vi "FAValuesXYZC.vi"(11 "Input":string[](array[string])) -> (3 "Output":string[][](array[string]))   [LabVIEW 2016, in "M1M3SupportEUI_Views.lvlib"]
uses:
  M1M3SupportEUI_Views.lvlib
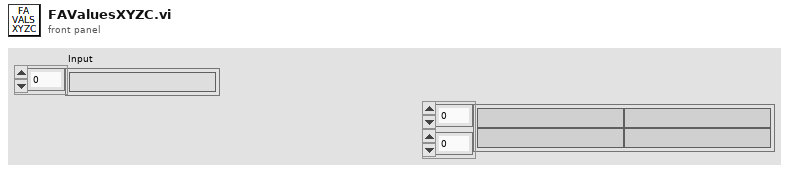
[diagram p1: front panel]
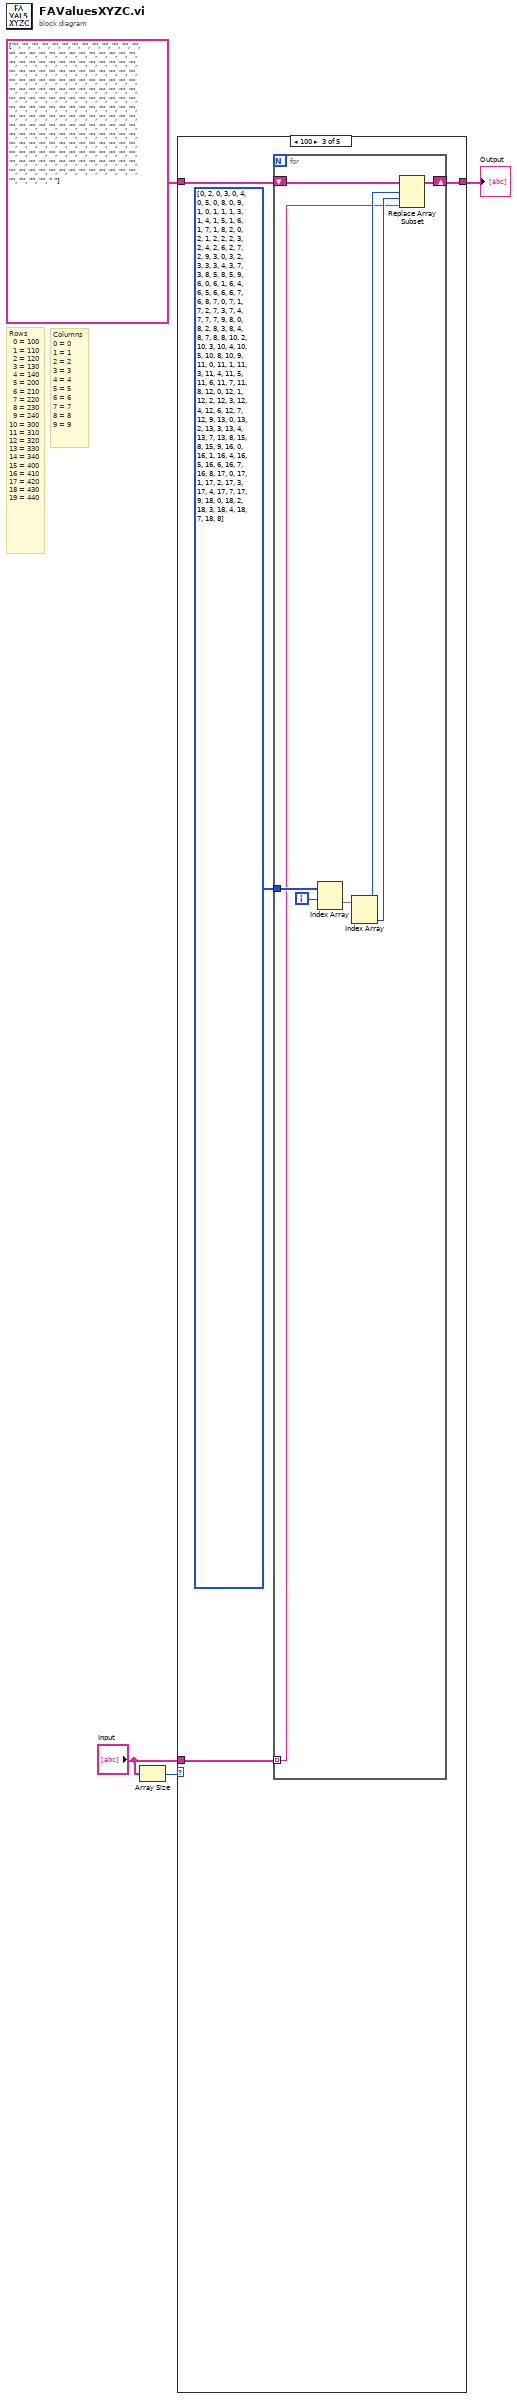
[diagram p0: block diagram]
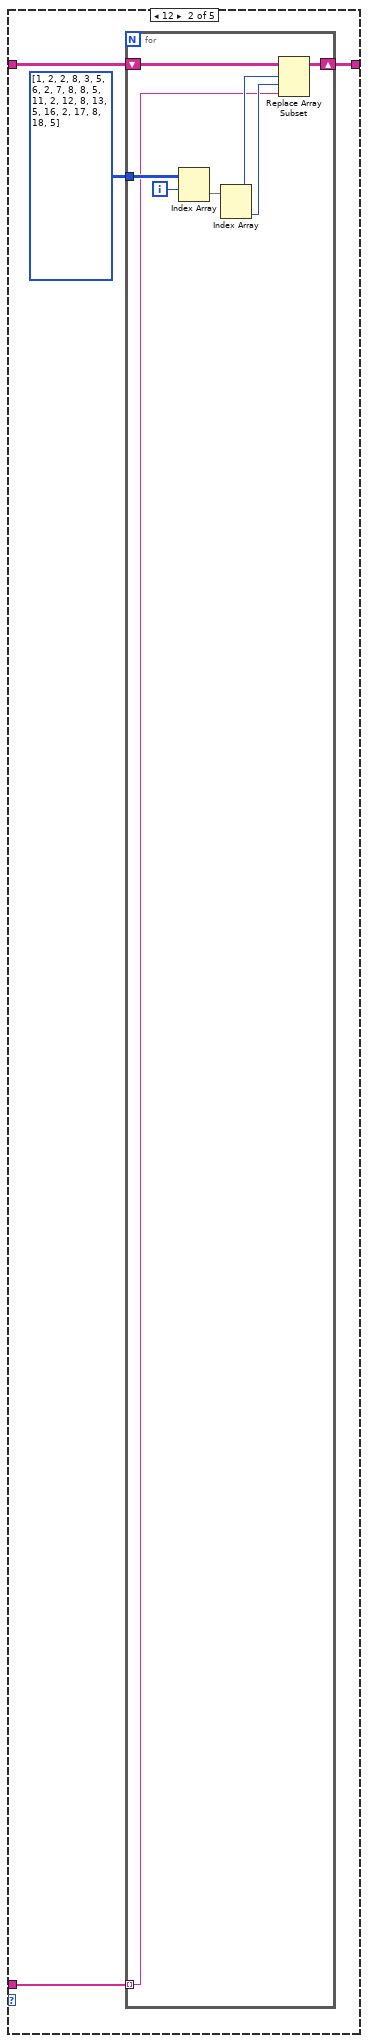
[diagram p3: hidden frame]
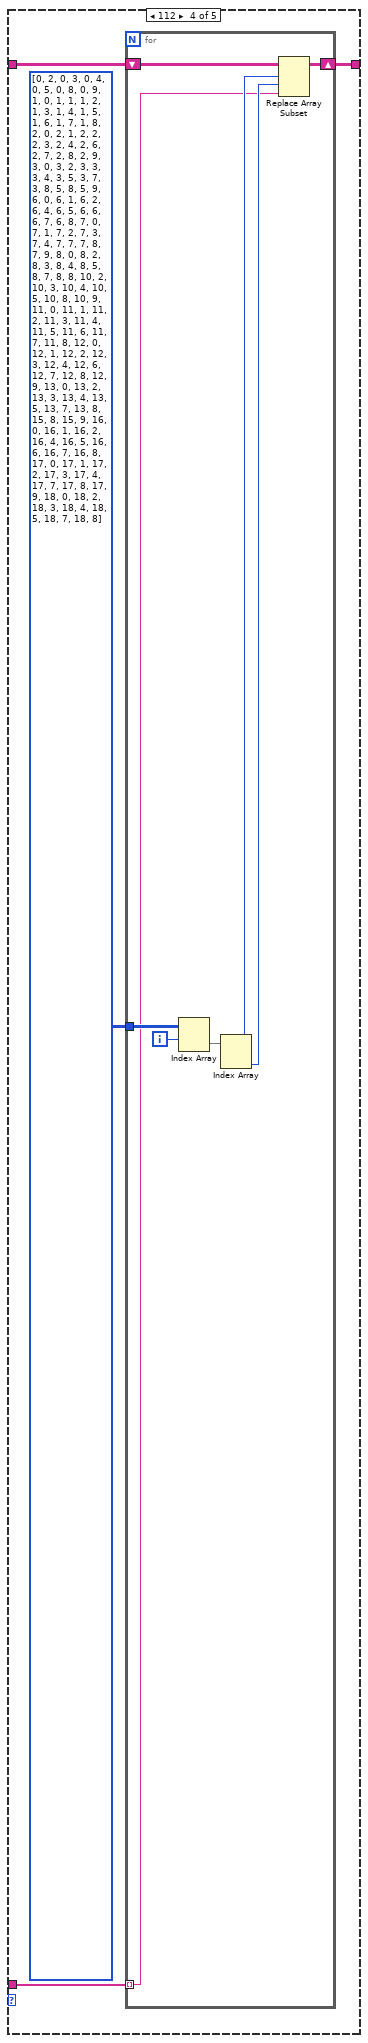
[diagram p4: hidden frame]
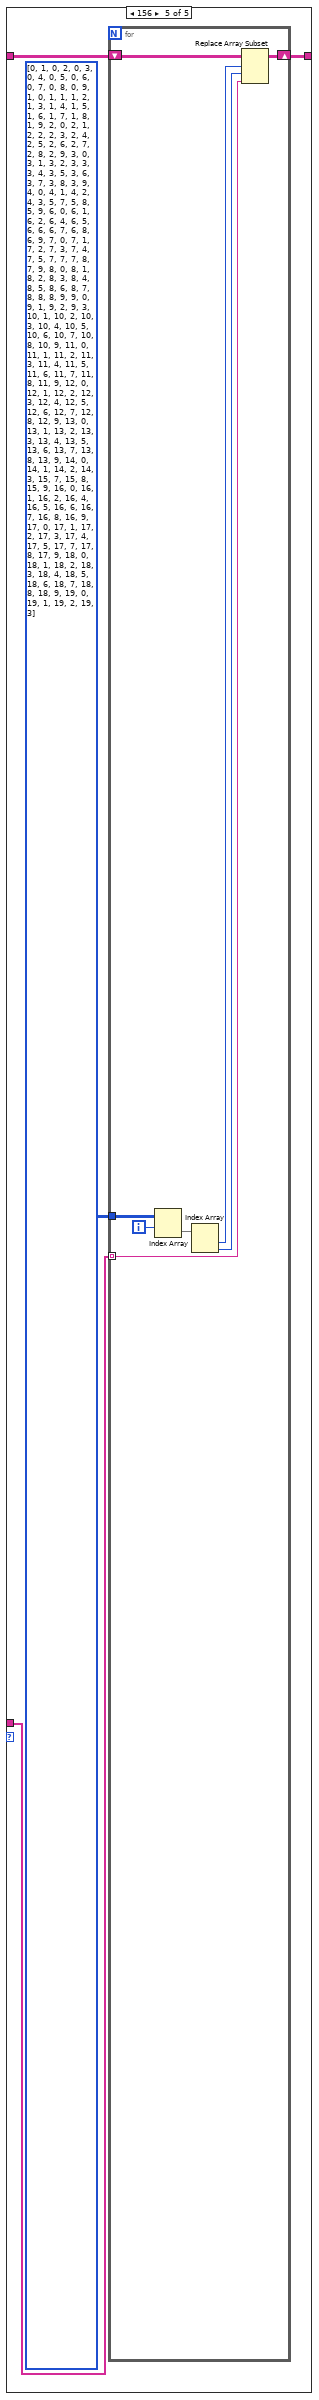
[diagram p5: hidden frame]
diagram:
  # "Columns\n0 = 0\n1 = 1\n2 = 2\n3 = 3\n4 = 4\n5 = 5\n6 = 6\n7 = 7\n8 = 8\n9 = 9"
  # "Rows\n  0 = 100\n  1 = 110\n  2 = 120\n  3 = 130\n  4 = 140\n  5 = 200\n  6 = 210\n  7 = 220\n  8 = 230\n  9 = 240\n10 = 300\n11 = 310\n12 = 320\n13 = 330\n14 = 340\n15 = 400\n16 = 410\n17 = 420\n18 = 430\n19 = 440"
  n1 = Array Size(array="Input") -> (size(s)=w4:i32)
  n2 = case shown="100" w4 {
    tunnel: "Input" -> [_ w7 w19 w31 w43]
    tunnel: string[][] [["", "", "", "", "", "", "", "", "", ""], ["", "", "", "", "", "", "", "", "", ""], ["", "", "", "", "", "", "", "", "", ""], ["", "", "", "", "", "", "", "", "", ""], ["", "", "", "", "", "", "", "", "", ""], ["", "", "", "", "", "", "", "", "", ""], ["", "", "", "", "", "", "", "", "", ""], ["", "", "", "", "", "", "", "", "", ""], ["", "", "", "", "", "", "", "", "", ""], ["", "", "", "", "", "", "", "", "", ""], ["", "", "", "", "", "", "", "", "", ""], ["", "", "", "", "", "", "", "", "", ""], ["", "", "", "", "", "", "", "", "", ""], ["", "", "", "", "", "", "", "", "", ""], ["", "", "", "", "", "", "", "", "", ""], ["", "", "", "", "", "", "", "", "", ""], ["", "", "", "", "", "", "", "", "", ""], ["", "", "", "", "", "", "", "", "", ""], ["", "", "", "", "", "", "", "", "", ""], ["", "", "", "", "", "", "", "", "", " "]] -> [w5 w9 w21 w33 w45]
    tunnel: [w5 w6 w18 w30 w42] -> w1
    frame 0, Default {
    }
    frame 12 {
      n3 = for {
        shift-right: [w16] -> w6
        shift-left: w9 -> [w17]
        tunnel: i32[][] [[1, 2], [2, 8], [3, 5], [6, 2], [7, 8], [8, 5], [11, 2], [12, 8], [13, 5], [16, 2], [17, 8], [18, 5]] -> [w15]
        tunnel: w7 -> [w10] mode=indexing
        i -> [w14]
        n4 = Index Array(array=w15, index (row)=w14) -> (element=w13:i32[])  [unwired: 1 in]
        n5 = Index Array(array=w13) -> (element #1=w12:i32, element #2=w11:i32)  [unwired: 2 in]
        n6 = Replace Array Subset(array=w17, new element=w10, index (row)=w12, index (col)=w11) -> (w16:string[][])
      }
    }
    frame 100 {
      n7 = for {
        shift-right: [w28] -> w18
        shift-left: w21 -> [w29]
        tunnel: i32[][] [[0, 2], [0, 3], [0, 4], [0, 5], [0, 8], [0, 9], [1, 0], [1, 1], [1, 3], [1, 4], [1, 5], [1, 6], [1, 7], [1, 8], [2, 0], [2, 1], [2, 2], [2, 3], [2, 4], [2, 6], [2, 7], [2, 9], [3, 0], [3, 2], [3, 3], [3, 4], [3, 7], [3, 8], [5, 8], [5, 9], [6, 0], [6, 1], [6, 4], [6, 5], [6, 6], [6, 7], [6, 8], [7, 0], [7, 1], [7, 2], [7, 3], [7, 4], [7, 7], [7, 9], [8, 0], [8, 2], [8, 3], [8, 4], [8, 7], [8, 8], [10, 2], [10, 3], [10, 4], [10, 5], [10, 8], [10, 9], [11, 0], [11, 1], [11, 3], [11, 4], [11, 5], [11, 6], [11, 7], [11, 8], [12, 0], [12, 1], [12, 2], [12, 3], [12, 4], [12, 6], [12, 7], [12, 9], [13, 0], [13, 2], [13, 3], [13, 4], [13, 7], [13, 8], [15, 8], [15, 9], [16, 0], [16, 1], [16, 4], [16, 5], [16, 6], [16, 7], [16, 8], [17, 0], [17, 1], [17, 2], [17, 3], [17, 4], [17, 7], [17, 9], [18, 0], [18, 2], [18, 3], [18, 4], [18, 7], [18, 8]] -> [w27]
        tunnel: w19 -> [w22] mode=indexing
        i -> [w26]
        n8 = Index Array(array=w27, index (row)=w26) -> (element=w25:i32[])  [unwired: 1 in]
        n9 = Index Array(array=w25) -> (element #1=w24:i32, element #2=w23:i32)  [unwired: 2 in]
        n10 = Replace Array Subset(array=w29, new element=w22, index (row)=w24, index (col)=w23) -> (w28:string[][])
      }
    }
    frame 112 {
      n11 = for {
        shift-right: [w40] -> w30
        shift-left: w33 -> [w41]
        tunnel: i32[][] [[0, 2], [0, 3], [0, 4], [0, 5], [0, 8], [0, 9], [1, 0], [1, 1], [1, 2], [1, 3], [1, 4], [1, 5], [1, 6], [1, 7], [1, 8], [2, 0], [2, 1], [2, 2], [2, 3], [2, 4], [2, 6], [2, 7], [2, 8], [2, 9], [3, 0], [3, 2], [3, 3], [3, 4], [3, 5], [3, 7], [3, 8], [5, 8], [5, 9], [6, 0], [6, 1], [6, 2], [6, 4], [6, 5], [6, 6], [6, 7], [6, 8], [7, 0], [7, 1], [7, 2], [7, 3], [7, 4], [7, 7], [7, 8], [7, 9], [8, 0], [8, 2], [8, 3], [8, 4], [8, 5], [8, 7], [8, 8], [10, 2], [10, 3], [10, 4], [10, 5], [10, 8], [10, 9], [11, 0], [11, 1], [11, 2], [11, 3], [11, 4], [11, 5], [11, 6], [11, 7], [11, 8], [12, 0], [12, 1], [12, 2], [12, 3], [12, 4], [12, 6], [12, 7], [12, 8], [12, 9], [13, 0], [13, 2], [13, 3], [13, 4], [13, 5], [13, 7], [13, 8], [15, 8], [15, 9], [16, 0], [16, 1], [16, 2], [16, 4], [16, 5], [16, 6], [16, 7], [16, 8], [17, 0], [17, 1], [17, 2], [17, 3], [17, 4], [17, 7], [17, 8], [17, 9], [18, 0], [18, 2], [18, 3], [18, 4], [18, 5], [18, 7], [18, 8]] -> [w39]
        tunnel: w31 -> [w34] mode=indexing
        i -> [w38]
        n12 = Index Array(array=w39, index (row)=w38) -> (element=w37:i32[])  [unwired: 1 in]
        n13 = Index Array(array=w37) -> (element #1=w36:i32, element #2=w35:i32)  [unwired: 2 in]
        n14 = Replace Array Subset(array=w41, new element=w34, index (row)=w36, index (col)=w35) -> (w40:string[][])
      }
    }
    frame 156 {
      n15 = for {
        shift-right: [w52] -> w42
        shift-left: w45 -> [w53]
        tunnel: i32[][] [[0, 1], [0, 2], [0, 3], [0, 4], [0, 5], [0, 6], [0, 7], [0, 8], [0, 9], [1, 0], [1, 1], [1, 2], [1, 3], [1, 4], [1, 5], [1, 6], [1, 7], [1, 8], [1, 9], [2, 0], [2, 1], [2, 2], [2, 3], [2, 4], [2, 5], [2, 6], [2, 7], [2, 8], [2, 9], [3, 0], [3, 1], [3, 2], [3, 3], [3, 4], [3, 5], [3, 6], [3, 7], [3, 8], [3, 9], [4, 0], [4, 1], [4, 2], [4, 3], [5, 7], [5, 8], [5, 9], [6, 0], [6, 1], [6, 2], [6, 4], [6, 5], [6, 6], [6, 7], [6, 8], [6, 9], [7, 0], [7, 1], [7, 2], [7, 3], [7, 4], [7, 5], [7, 7], [7, 8], [7, 9], [8, 0], [8, 1], [8, 2], [8, 3], [8, 4], [8, 5], [8, 6], [8, 7], [8, 8], [8, 9], [9, 0], [9, 1], [9, 2], [9, 3], [10, 1], [10, 2], [10, 3], [10, 4], [10, 5], [10, 6], [10, 7], [10, 8], [10, 9], [11, 0], [11, 1], [11, 2], [11, 3], [11, 4], [11, 5], [11, 6], [11, 7], [11, 8], [11, 9], [12, 0], [12, 1], [12, 2], [12, 3], [12, 4], [12, 5], [12, 6], [12, 7], [12, 8], [12, 9], [13, 0], [13, 1], [13, 2], [13, 3], [13, 4], [13, 5], [13, 6], [13, 7], [13, 8], [13, 9], [14, 0], [14, 1], [14, 2], [14, 3], [15, 7], [15, 8], [15, 9], [16, 0], [16, 1], [16, 2], [16, 4], [16, 5], [16, 6], [16, 7], [16, 8], [16, 9], [17, 0], [17, 1], [17, 2], [17, 3], [17, 4], [17, 5], [17, 7], [17, 8], [17, 9], [18, 0], [18, 1], [18, 2], [18, 3], [18, 4], [18, 5], [18, 6], [18, 7], [18, 8], [18, 9], [19, 0], [19, 1], [19, 2], [19, 3]] -> [w51]
        tunnel: w43 -> [w46] mode=indexing
        i -> [w50]
        n16 = Index Array(array=w51, index (row)=w50) -> (element=w49:i32[])  [unwired: 1 in]
        n17 = Index Array(array=w49) -> (element #1=w48:i32, element #2=w47:i32)  [unwired: 2 in]
        n18 = Replace Array Subset(array=w53, new element=w46, index (row)=w48, index (col)=w47) -> (w52:string[][])
      }
    }
  }
  "Output" <- w1
